vi "Read_Stage_Variant.vi"(8 "error in (no error)":errorcluster, 9 "Variant":variant) -> (0 "error out":errorcluster, 2 "Channels":u8, 3 "Output Voltage":dbl)   [LabVIEW 2023]
uses:
  <userlib>/_OpenG.lib/lvdata/lvdata.llb/openg_variant.lvlib
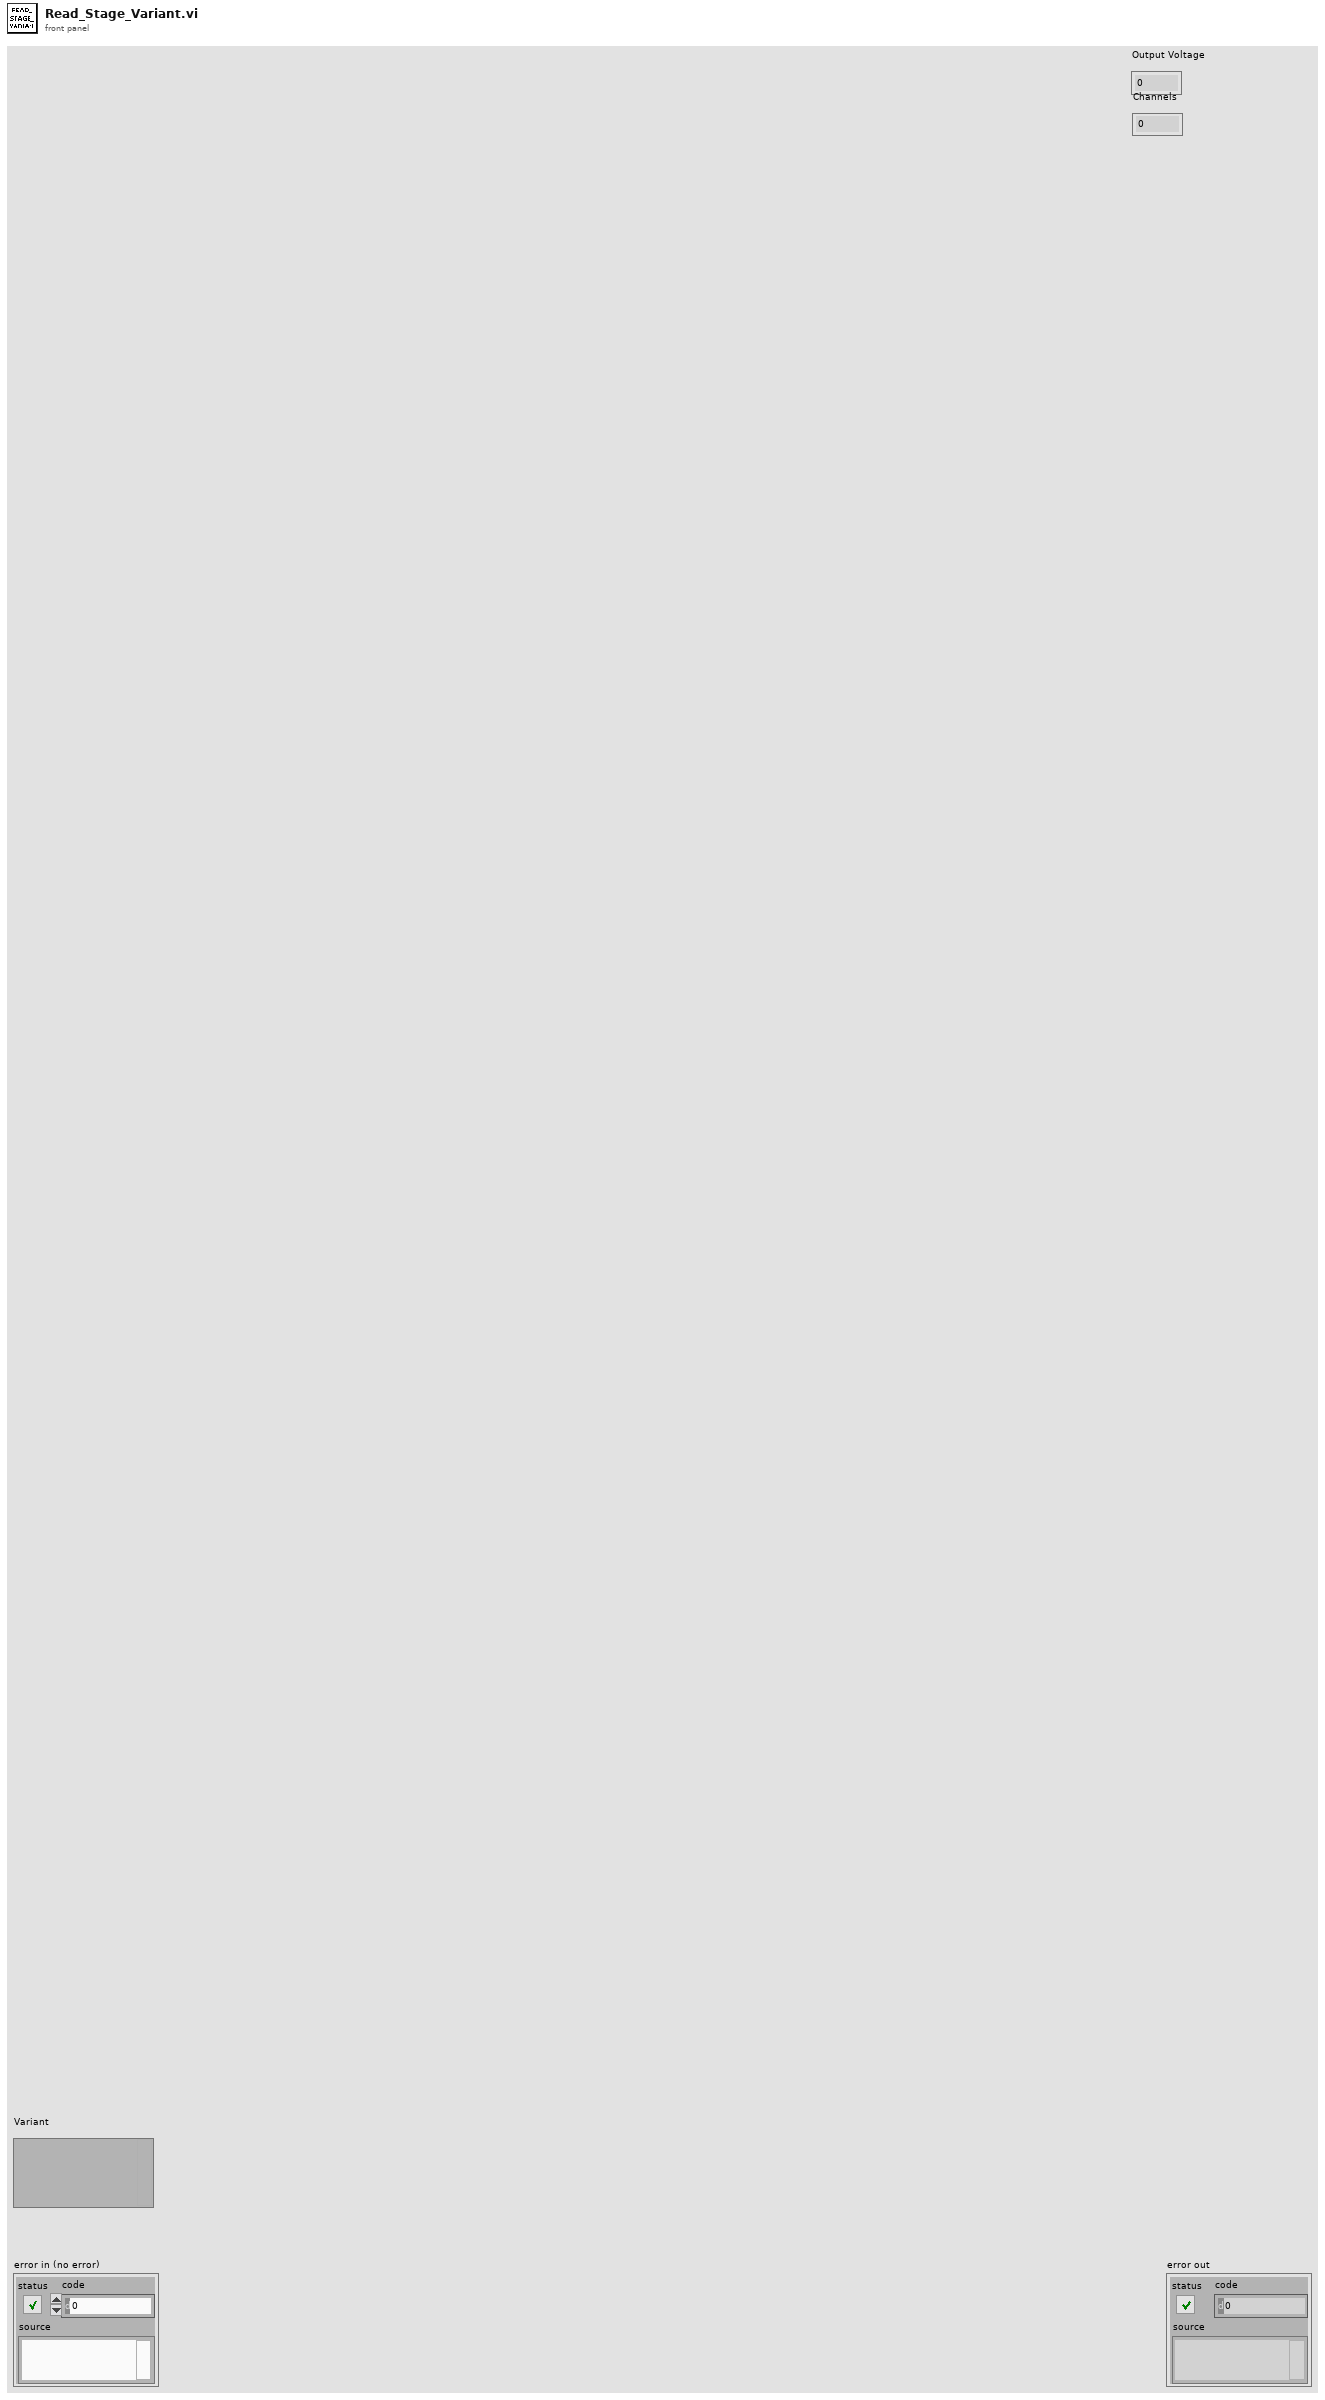
[diagram p1: front panel]
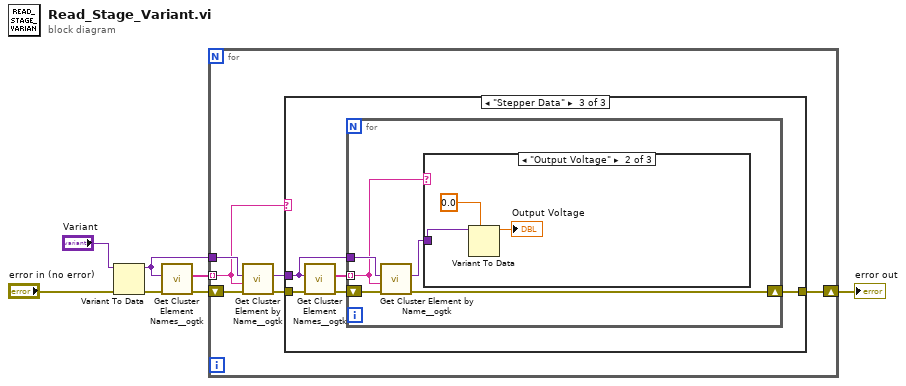
[diagram p0: block diagram]
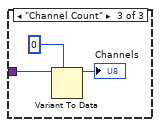
[diagram p5: hidden frame]
diagram:
  n1 = Variant To Data(error in="error in (no error)", Variant="Variant") -> (data=w4:variant, error out=w6:errorcluster)  [unwired: 1 in]
  n2 = call <userlib>:"Get Cluster Element Names__ogtk.vi"("error in (no error)"=w6, "Cluster"=w4) -> ("error out"=w5:errorcluster, "Element Names"=w3:string[])  [unwired: 8 in]
  n3 = for {
    tunnel: w3 -> [w12] mode=indexing
    tunnel: w4 -> [w13]
    shift-right: [w8] -> w7
    shift-left: w5 -> [w9]
    n4 = call <userlib>:"Get Cluster Element by Name__ogtk.vi"("error in (no error)"=w9, "Element Name"=w12, "Cluster"=w13) -> ("error out"=w10:errorcluster, "VElement"=w11:variant)  [unwired: 6 in, 1 out]
    n5 = case shown="\"Stepper Data\"" w12 {
      tunnel: w11 -> [_ _ w19]
      tunnel: w10 -> [w14 w15 w18]
      tunnel: [w14 w15 w16] -> w8
      frame "False", Default {
      }
      frame "InstrData" {
      }
      frame "Stepper Data" {
        n6 = call <userlib>:"Get Cluster Element Names__ogtk.vi"("error in (no error)"=w18, "Cluster"=w19) -> ("error out"=w17:errorcluster, "Element Names"=w20:string[])  [unwired: 8 in]
        n7 = for {
          tunnel: w20 -> [w24] mode=indexing
          tunnel: w19 -> [w25]
          shift-right: [w21] -> w16
          shift-left: w17 -> [w22]
          n8 = call <userlib>:"Get Cluster Element by Name__ogtk.vi"("error in (no error)"=w22, "Element Name"=w24, "Cluster"=w25) -> ("error out"=w21:errorcluster, "VElement"=w23:variant)  [unwired: 6 in, 1 out]
          n9 = case shown="\"Output Voltage\"" w24 {
            tunnel: w23 -> [_ w28 w31]
            frame "False", Default {
            }
            frame "Output Voltage" {
              n10 = Variant To Data(type=0.0, Variant=w28) -> (data=→"Output Voltage":dbl)  [unwired: 1 in, 1 out]
            }
            frame "Channel Count" {
              n11 = Variant To Data(type=u8 0, Variant=w31) -> (data=→"Channels":u8)  [unwired: 1 in, 1 out]
            }
          }
        }
      }
    }
  }
  "error out" <- w7
